vi "Get Msg Attributes.vi"(11 "Actor Destroy Msg Strategy in":refnum<class "Actor Destroy Msg Strategy.lvclass">) -> ()   [LabVIEW 2021, in "Actor Destroy.lvlib" / "Actor Destroy Msg Strategy.lvclass"]
uses:
  Actor Destroy Msg Strategy.lvclass
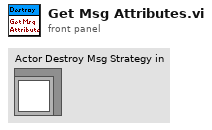
[diagram p1: front panel]
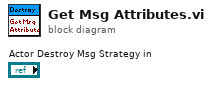
[diagram p0: block diagram]
diagram:
